vi "MARS_Dload_Config_param.vi"(8 "Error in":errorcluster, 10 "Integ_per":cluster{dbl, dbl}(slide) caption="Duration of Integration (us)" scale=0.0..10.0, 11 "VISA Resource name":refnum<visa-resource-name>) -> (0 "error out":errorcluster, 3 "VISA resource name out":refnum<visa-resource-name>)   [LabVIEW 2015]
uses:
  MARS_Global_var.vi
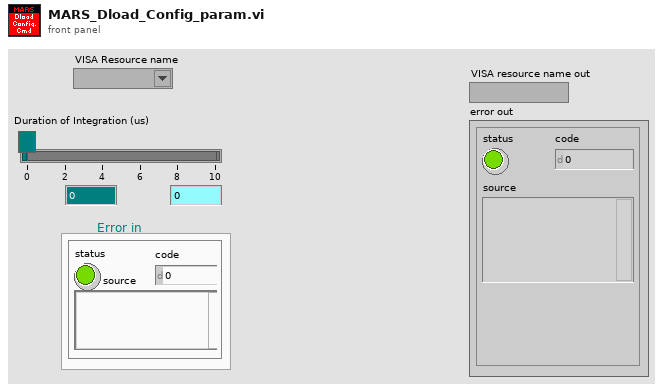
[diagram p1: front panel]
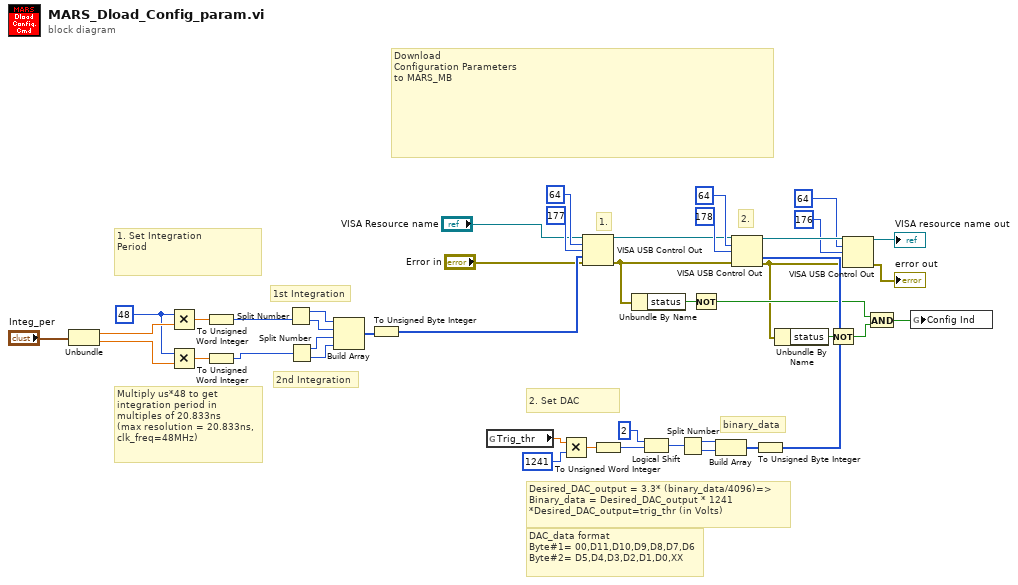
[diagram p0: block diagram]
diagram:
  w27 = u16 48 ("x")
  # "2."
  # "binary_data"
  # "1."
  # "DAC_data format\nByte#1= 00,D11,D10,D9,D8,D7,D6\nByte#2= D5,D4,D3,D2,D1,D0,XX"
  # "Desired_DAC_output = 3.3* (binary_data/4096)=>\nBinary_data = Desired_DAC_output * 1241\n*Desired_DAC_output=trig_thr (in Volts)"
  # "Multiply us*48 to get \nintegration period in \nmultiples of 20.833ns \n(max resolution = 20.833ns,\nclk_freq=48MHz)"
  # "2nd Integration"
  # "1st Integration"
  # "Download\nConfiguration Parameters\nto MARS_MB"
  # "1. Set Integration\nPeriod"
  # "2. Set DAC"
  n1 = Unbundle("Integ_per") -> (w28:dbl, w9:dbl)
  n2 = Multiply(x=w27, y=w28) -> (x*y=w26:dbl)
  n3 = Multiply(x=w27, y=w9) -> (x*y=w25:dbl)
  n4 = To Unsigned Word Integer(number=w26) -> (unsigned 16bit integer=w8:u16)
  n5 = To Unsigned Word Integer(number=w25) -> (unsigned 16bit integer=w7:u16)
  n6 = Split Number(x=w8) -> (hi(x)=w24:u8, lo(x)=w23:u8)
  n7 = Split Number(x=w7) -> (hi(x)=w21:u8, lo(x)=w22:u8)
  n8 = Build Array(w24, w23, w21, w22) -> (w20:u8[])
  n9 = To Unsigned Byte Integer(number=w20) -> (unsigned 8bit integer=w19:u8[])
  n10 = global read "MARS_Global_var.vi" "Trig_thr"() -> (w34:dbl)
  n11 = Multiply(x=w34, y=1241) -> (x*y=w32:dbl)
  n12 = VISA USB Control Out(0:"VISA Resource name", 5:i16 64 ("request type"), 7:i16 177 ("request type"), 9:w19, 11:"Error in") -> (4:w29:refnum<visa-resource-name>, 15:w17:errorcluster)  [unwired: 2 in]
  n13 = To Unsigned Word Integer(number=w32) -> (unsigned 16bit integer=w35:u16)
  n14 = Unbundle By Name(w17) -> ("status"=w16:bool)
  n15 = Logical Shift(y=i16 2, x=w35) -> (x << y=w37:u16)
  n16 = Split Number(x=w37) -> (hi(x)=w38:u8, lo(x)=w39:u8)
  n17 = Not(x=w16) -> (.not. x?=w15:bool)
  n18 = Build Array(w38, w39) -> (w40:u8[])
  n19 = To Unsigned Byte Integer(number=w40) -> (unsigned 8bit integer=w43:u8[])
  n20 = VISA USB Control Out(0:w29, 5:i16 64 ("request type"), 7:i16 178 ("request type"), 9:w43, 11:w17) -> (4:w6:refnum<visa-resource-name>, 15:w5:errorcluster)  [unwired: 2 in]
  n21 = Unbundle By Name(w5) -> ("status"=w14:bool)
  n22 = Not(x=w14) -> (.not. x?=w13:bool)
  n23 = VISA USB Control Out(0:w6, 5:i16 64 ("request type"), 7:i16 176 ("request type"), 11:w5) -> (4:→"VISA resource name out":refnum<visa-resource-name>, 15:→"error out":errorcluster)  [unwired: 3 in]
  n24 = And(x=w15, y=w13) -> (x .and. y?=w18:bool)
  n25 = global write "MARS_Global_var.vi" "Config Ind"(w18) -> ()
